vi "spin_map.vi"(4 "pos_y":dbl, 6 "pos_x":dbl, 7 "scale":dbl, 8 "spin":dbl(slide) scale=-1.0..1.0, 10 "x":dbl(slide) scale=-1.0..1.0, 11 "y":dbl(slide) scale=-1.0..1.0) -> (0 "mag":dbl, 3 "angle":dbl)   [LabVIEW 2023]
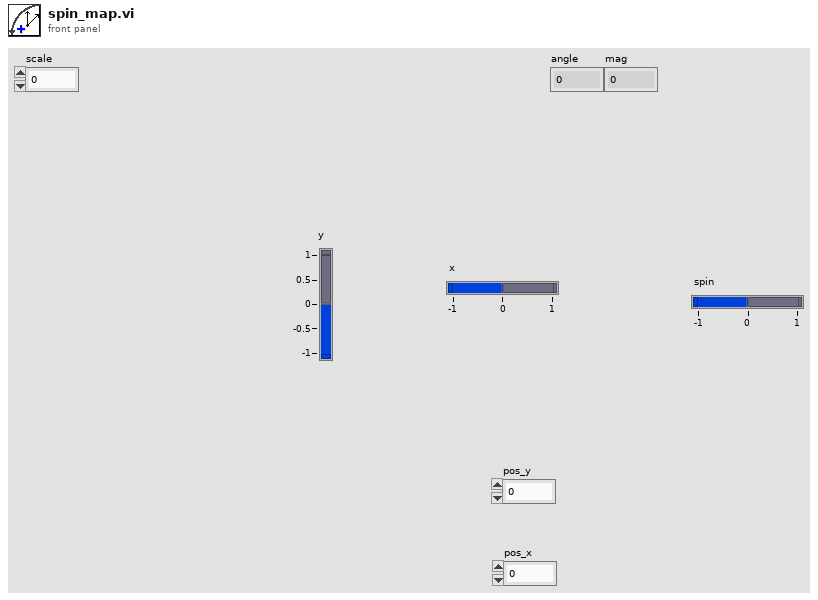
[diagram p1: front panel]
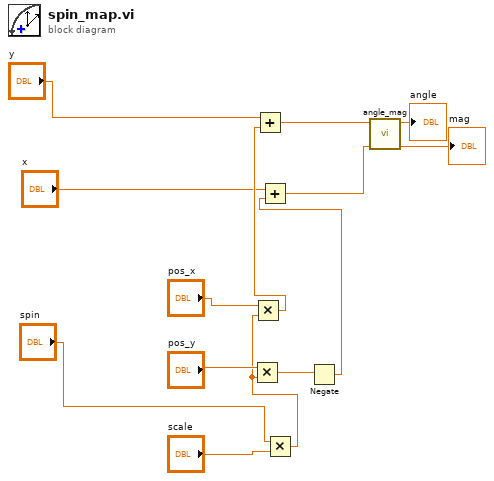
[diagram p0: block diagram]
diagram:
  n1 = Multiply(x="spin", y="scale") -> (x*y=w4:dbl)
  n2 = Multiply(x="pos_y", y=w4) -> (x*y=w12:dbl)
  n3 = Multiply(x="pos_x", y=w4) -> (x*y=w9:dbl)
  n4 = Add(x="y", y=w9) -> (x+y=w11:dbl)
  n5 = Negate(x=w12) -> (-x=w7:dbl)
  n6 = Add(x="x", y=w7) -> (x+y=w6:dbl)
  n7 = call "angle_mag.vi"("x"=w6, "y"=w11) -> ("mag"=→"mag":dbl, "angle"=→"angle":dbl)  [unwired: 8 in]
